vi "Check Status.vi"(8 "error in (no error)":errorcluster, 11 "Pulse Generator in":refnum<class "Pulse Generator.lvclass">) -> (0 "error out":errorcluster, 1 "Status":string, 2 "Ready?":bool, 3 "Pulse Generator out":refnum<class "Pulse Generator.lvclass">)   [LabVIEW 2009, in "Pulse Generator.lvclass"]
doc: "Checks if the instrument is powered on and updates its member data with the instrument's current status."
uses:
  Pulse Generator.lvclass
  Utility Classes/Scannable/Scannable.lvclass
  Pulse Generator.lvclass/Pulse Generator.ctl
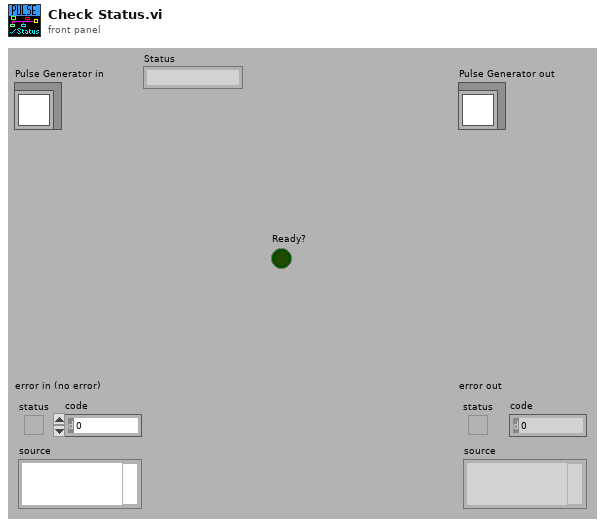
[diagram p1: front panel]
types:
  T1 = enum16{"Invalid", "Channel 1", "Channel 2", "Strobe"}
  T2 = enum16{"Immediate (Continuous Mode)", "Internal PLL", "External", "Manual"}
  T3 = enum32{"Continuous Pulsed", "Continuous Pattern", "Internal Triggered Pattern", "External Triggered Pulsed", "External Triggered Pattern", "Other"}
  T4 = cluster{"Value High":dbl[unit], "Value Low":dbl[unit], "Value High":dbl[unit], "Value Low":dbl[unit]}
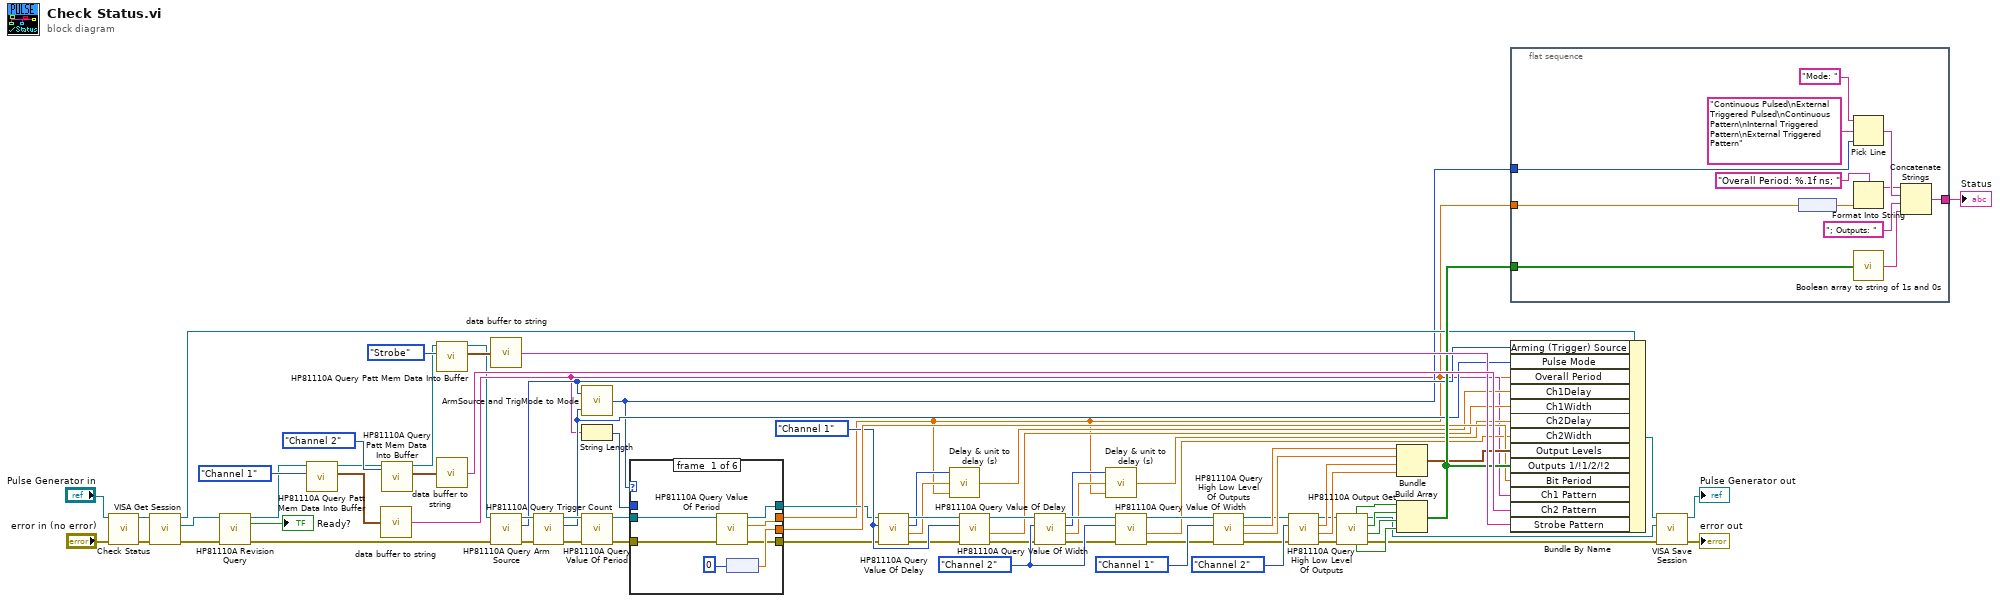
[diagram p0: block diagram]
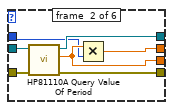
[diagram p2: hidden frame]
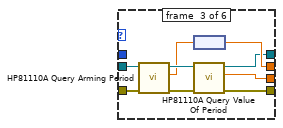
[diagram p3: hidden frame]
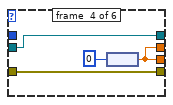
[diagram p4: hidden frame]
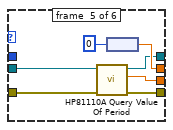
[diagram p5: hidden frame]
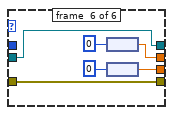
[diagram p6: hidden frame]
diagram:
  w30 = enum16{"Invalid", "Channel 1", "Channel 2"}."Channel 2" ("Channel (1:Channel 1)")
  w31 = enum16{"Invalid", "Channel 1", "Channel 2"}."Channel 1" ("Channel (1:Channel 1)")
  n1 = call-parent "Check Status.vi"("error in (no error)"="error in (no error)", "Instrument in"="Pulse Generator in") -> ("error out"=w69:errorcluster, "Instrument out"=w70:refnum<class "Pulse Generator.lvclass">)  [unwired: 8 out]
  n2 = call-dynamic "VISA Get Session.vi"("error in (no error)"=w69, "Instrument.lvclass in"=w70) -> ("error out"=w66:errorcluster, "VISA Resource Name"=w65:refnum<visa-resource-name>, "Instrument.lvclass out"=w40:refnum<class "Pulse Generator.lvclass">)  [unwired: 7 out]
  n3 = call "HP81110A Revision Query.vi"("VISA session"=w65, "error in (no error)"=w66) -> ("dup VISA session"=w11:refnum<visa-resource-name>, "Ready?"=→"Ready?":bool, "error out"=w19:errorcluster)  [unwired: 11 out]
  n4 = call "HP81110A Query Patt Mem Data Into Buffer.vi"("Channel (1:Channel 1)"=T1."Channel 1", "VISA session"=w11) -> ("output pattern"=w51:digitaldata, "dup VISA session"=w53:refnum<visa-resource-name>)  [unwired: 1 in, 7 out]
  n5 = call "data buffer to string.vi"("output pattern"=w51) -> ("initial string"=w14:string)
  n6 = call "HP81110A Query Patt Mem Data Into Buffer.vi"("Channel (1:Channel 1)"=T1."Channel 2", "VISA session"=w53) -> ("output pattern"=w50:digitaldata, "dup VISA session"=w52:refnum<visa-resource-name>)  [unwired: 1 in, 7 out]
  n7 = call "HP81110A Query Patt Mem Data Into Buffer.vi"("Channel (1:Channel 1)"=T1."Strobe", "VISA session"=w52) -> ("output pattern"=w49:digitaldata, "dup VISA session"=w10:refnum<visa-resource-name>)  [unwired: 1 in, 7 out]
  n8 = call "data buffer to string.vi"("output pattern"=w50) -> ("initial string"=w48:string)
  n9 = call "data buffer to string.vi"("output pattern"=w49) -> ("initial string"=w47:string)
  n10 = call "HP81110A Query Arm Source.vi"("error in (no error)"=w19, "VISA session"=w10) -> ("error out"=w18:errorcluster, "Arming (Trigger) Source (0:Internal PLL)"=w36:T2, "dup VISA session"=w42:refnum<visa-resource-name>)  [unwired: 7 out]
  n11 = call "HP81110A Query Trigger Count.vi"("error in (no error)"=w18, "VISA session"=w42) -> ("error out"=w17:errorcluster, "Pulse Mode"=w35:enum16{"Pulses", "Pattern"}, "dup VISA session"=w41:refnum<visa-resource-name>)  [unwired: 7 out]
  n12 = call "ArmSource and TrigMode to Mode.vi"("Pulse Mode"=w35, "Arming (Trigger) Source (0:Internal PLL)"=w36) -> ("Modes (changes immediately)"=w15:T3)
  n13 = String Length(string=w14) -> (length=w13:i32)
  n14 = call "HP81110A Query Value Of Period.vi"("error in (no error)"=w17, "VISA session"=w41) -> ("error out"=w16:errorcluster, "dup VISA session"=w37:refnum<visa-resource-name>)  [unwired: 1 in, 7 out]
  n15 = case shown="\"External Triggered Pattern\"" w15 {
    tunnel: [w82 w89 w95 w102 w108 w113] -> w9
    tunnel: [w81 w90 w96 w102 w109 w114] -> w38
    tunnel: w37 -> [w80 w88 w94 w101 w107 w112]
    tunnel: [w79 w87 w93 w100 w106 w111] -> w8
    tunnel: [w78 w86 w92 w101 w105 w112] -> w28
    tunnel: w16 -> [w77 w85 w91 w100 w104 w111]
    tunnel: w13 -> [_ w84 _ _ _ _]
    frame #0 {
      n16 = call "HP81110A Query Value Of Period.vi"("error in (no error)"=w77, "VISA session"=w80) -> ("error out"=w79:errorcluster, "Period Value"=w82:dbl[unit], "dup VISA session"=w78:refnum<visa-resource-name>)  [unwired: 7 out]
      n17 = node(0) -> (w81:dbl[unit])
    }
    frame #1 {
      n18 = call "HP81110A Query Value Of Period.vi"("error in (no error)"=w85, "VISA session"=w88) -> ("error out"=w87:errorcluster, "Period Value"=w90:dbl[unit], "dup VISA session"=w86:refnum<visa-resource-name>)  [unwired: 7 out]
      n19 = Multiply(x=w90, y=w84) -> (x*y=w89:dbl[unit])
    }
    frame #2 {
      n20 = call "HP81110A Query Arming Period.vi"("error in (no error)"=w91, "VISA session"=w94) -> ("error out"=w99:errorcluster, "Period Value (Sec)"=w97:dbl, "dup VISA session"=w98:refnum<visa-resource-name>)  [unwired: 7 out]
      n21 = node(w97) -> (w95:dbl[unit])
      n22 = call "HP81110A Query Value Of Period.vi"("error in (no error)"=w99, "VISA session"=w98) -> ("error out"=w93:errorcluster, "Period Value"=w96:dbl[unit], "dup VISA session"=w92:refnum<visa-resource-name>)  [unwired: 7 out]
    }
    frame #3 {
      n23 = node(0) -> (w102:dbl[unit])
    }
    frame #4 {
      n24 = call "HP81110A Query Value Of Period.vi"("error in (no error)"=w104, "VISA session"=w107) -> ("error out"=w106:errorcluster, "Period Value"=w109:dbl[unit], "dup VISA session"=w105:refnum<visa-resource-name>)  [unwired: 7 out]
      n25 = node(0) -> (w108:dbl[unit])
    }
    frame #5 {
      n26 = node(0) -> (w113:dbl[unit])
      n27 = node(0) -> (w114:dbl[unit])
    }
  }
  n28 = call "HP81110A Query Value Of Delay.vi"("error in (no error)"=w8, "Channel (1:Channel 1)"=w31, "VISA session"=w28) -> ("error out"=w7:errorcluster, "Delay Value"=w26:dbl, "Delay Unit"=w27:u16, "dup VISA session"=w32:refnum<visa-resource-name>)  [unwired: 5 out]
  n29 = call "Delay & unit to delay (s).vi"("OverallPeriod"=w9, "Delay Value"=w26, "Delay Unit"=w27) -> ("Delay (s)"=w25:dbl[unit])
  n30 = call "HP81110A Query Value Of Width.vi"("error in (no error)"=w7, "Channel (1:Channel 1)"=w31, "VISA session"=w32) -> ("error out"=w6:errorcluster, "Width Value (Sec)"=w24:dbl[unit], "dup VISA session"=w34:refnum<visa-resource-name>)  [unwired: 6 out]
  n31 = call "HP81110A Query Value Of Delay.vi"("error in (no error)"=w6, "Channel (1:Channel 1)"=w30, "VISA session"=w34) -> ("error out"=w5:errorcluster, "Delay Value"=w22:dbl, "Delay Unit"=w23:u16, "dup VISA session"=w33:refnum<visa-resource-name>)  [unwired: 5 out]
  n32 = call "Delay & unit to delay (s).vi"("OverallPeriod"=w9, "Delay Value"=w22, "Delay Unit"=w23) -> ("Delay (s)"=w21:dbl[unit])
  n33 = call "HP81110A Query Value Of Width.vi"("error in (no error)"=w5, "Channel (1:Channel 1)"=w30, "VISA session"=w33) -> ("error out"=w4:errorcluster, "Width Value (Sec)"=w20:dbl[unit], "dup VISA session"=w29:refnum<visa-resource-name>)  [unwired: 6 out]
  n34 = call "HP81110A Query High Low Level Of Outputs.vi"("error in (no error)"=w4, "Channel (1:Channel 1)"=enum16{"Invalid", "Channel 1", "Channel 2"}."Channel 1", "VISA session"=w29) -> ("error out"=w3:errorcluster, "Value Low"=w62:dbl[unit], "Value High"=w63:dbl[unit], "dup VISA session"=w44:refnum<visa-resource-name>)  [unwired: 1 in, 4 out]
  n35 = call "HP81110A Query High Low Level Of Outputs.vi"("error in (no error)"=w3, "Channel (1:Channel 1)"=enum16{"Invalid", "Channel 1", "Channel 2"}."Channel 2", "VISA session"=w44) -> ("error out"=w2:errorcluster, "Value Low"=w60:dbl[unit], "Value High"=w61:dbl[unit], "dup VISA session"=w43:refnum<visa-resource-name>)  [unwired: 1 in, 4 out]
  n36 = call "HP81110A Output Get.vi"("error in (no error)"=w2, "VISA session"=w43) -> ("error out"=w1:errorcluster, "output2OUT"=w73:bool, "notoutput1OUT"=w72:bool, "dup VISA session"=w12:refnum<visa-resource-name>, "notoutput2OUT"=w74:bool, "output1OUT"=w71:bool)  [unwired: 4 out]
  n37 = Bundle("Value High"=w63, "Value Low"=w62, "Value High"=w61, "Value Low"=w60) -> (w45:T4)  [unwired: 1 out]
  n38 = Build Array(w71, w72, w73, w74) -> (w46:bool[])
  n39 = flat-sequence {
    tunnel: w46 -> [w119]
    tunnel: w9 -> [w123]
    tunnel: [w122] -> w39
    tunnel: w15 -> [w121]
    frame #0 {
      n40 = node(w123) -> (w127:dbl)
      n41 = Pick Line(string ("")="Mode: ", multi-line string="Continuous Pulsed\nExternal Triggered Pulsed\nContinuous Pattern\nInternal Triggered Pattern\nExternal Triggered Pattern", line index=w121) -> (output string=w125:string)
      n42 = Format Into String(format string="Overall Period: %.1f ns; ", w127) -> (resulting string=w124:string)  [unwired: 2 in, 1 out]
      n43 = call "Boolean array to string of 1s and 0s.vi"("Array"=w119) -> ("String"=w118:string)
      n44 = Concatenate Strings(w124, w125, "; Outputs: ", w118) -> (w122:string)
    }
  }
  n45 = Bundle By Name(cluster=w40, "Arming (Trigger) Source"=w36, "Pulse Mode"=w35, "Overall Period"=w9, "Ch1Delay"=w25, "Ch1Width"=w24, "Ch2Delay"=w21, "Ch2Width"=w20, "Output Levels"=w45, "Outputs 1/!1/2/!2"=w46, "Bit Period"=w38, "Ch1 Pattern"=w14, "Ch2 Pattern"=w48, "Strobe Pattern"=w47) -> (w57:refnum<class "Pulse Generator.lvclass">)
  n46 = call-dynamic "VISA Save Session.vi"("error in (no error)"=w1, "VISA Resource Name"=w12, "Instrument.lvclass in"=w57) -> ("error out"=→"error out":errorcluster, "Instrument.lvclass out"=→"Pulse Generator out":refnum<class "Pulse Generator.lvclass">)  [unwired: 7 out]
  "Status" <- w39
